vi "Validate Index.vi"(8 "error in (no error)":errorcluster, 11 "Indexing Test Finder in":refnum<class "Indexing Test Finder.lvclass">) -> (0 "error out":errorcluster, 3 "Indexing Test Finder out":refnum<class "Indexing Test Finder.lvclass">)   [LabVIEW 2020, in "Indexing Test Finder.lvclass"]
uses:
  Indexing Test Finder.lvclass
  Indexing Test Finder.lvclass/Indexing Test Finder.ctl
  TypeDefs/Index Item.ctl
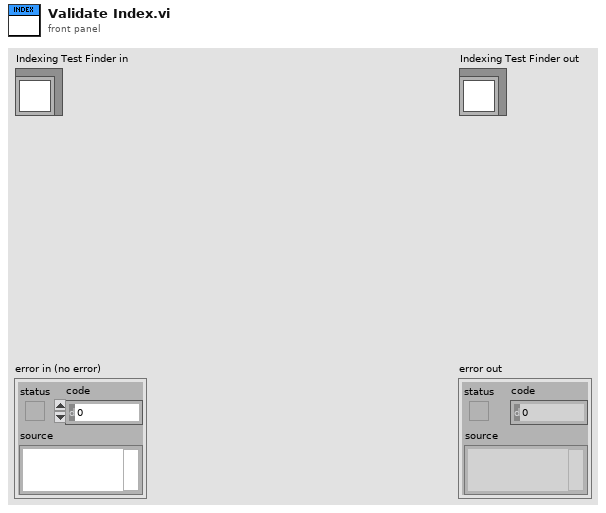
[diagram p1: front panel]
types:
  T1 = typedef "Indexing Test Finder.lvclass/Index Item.ctl" = cluster{"Dynamic Methods":map{string, path}, "Static Methods":map{string, path}, "Signature":string}
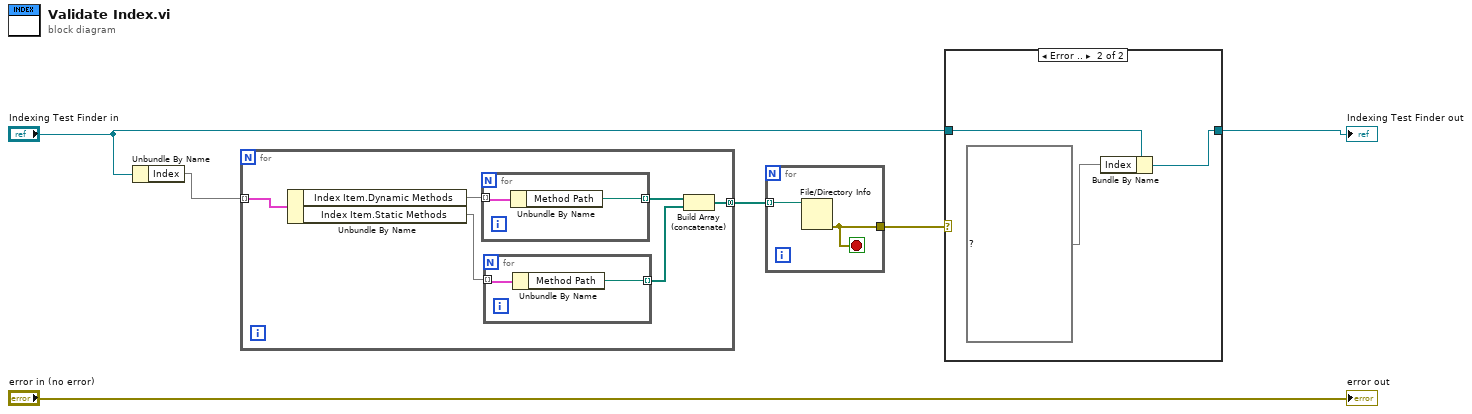
[diagram p0: block diagram]
diagram:
  n1 = Unbundle By Name("Indexing Test Finder in") -> ("Index"=w5:map{path, T1})
  n2 = for {
    tunnel: w5 -> [w12] mode=indexing
    tunnel: [w7] -> w4 mode=concatenating
    n3 = Unbundle By Name(w12) -> ("Index Item.Dynamic Methods"=w11:map{string, path}, "Index Item.Static Methods"=w10:map{string, path})
    n4 = for {
      tunnel: w11 -> [w16] mode=indexing
      tunnel: [w15] -> w9 mode=indexing
      n5 = Unbundle By Name(w16) -> ("Method Path"=w15:path)
    }
    n6 = for {
      tunnel: w10 -> [w14] mode=indexing
      tunnel: [w13] -> w8 mode=indexing
      n7 = Unbundle By Name(w14) -> ("Method Path"=w13:path)
    }
    n8 = Build Array (concatenate)(w9, w8) -> (w7:path[])
  }
  n9 = for {
    tunnel: w4 -> [w18] mode=indexing
    tunnel: [w17] -> w1
    stop <- w17 stop-if-true
    n10 = File/Directory Info(path=w18) -> (error out=w17:errorcluster)  [unwired: 1 in, 6 out]
  }
  n11 = case shown="Error .." w1 {
    tunnel: [w19 w20] -> w3
    tunnel: "Indexing Test Finder in" -> [w19 w22]
    frame No Error {
    }
    frame Error {
      n12 = Bundle By Name(cluster=w22, "Index"=map{path, T1} {}) -> (w20:refnum<class "Indexing Test Finder.lvclass">)
    }
  }
  "Indexing Test Finder out" <- w3
  "error out" <- "error in (no error)"
